vi "niDTS BT INSTR TX UTIL Average Type.vi"(7 "Type In":enum16{"RMS", "LOG", "SCALAR", "MAX", "MIN"}(ring)) -> (8 "Type Out":enum16{"RMS", "LOG", "SCALar", "MAX", "MIN"}(ring))   [LabVIEW 2015, in "niDTS BT.lvlib" / "niDTS BT INSTR TX.lvclass"]
uses:
  niDTS BT INSTR TX.lvclass
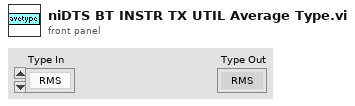
[diagram p1: front panel]
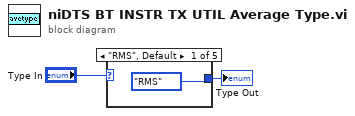
[diagram p0: block diagram]
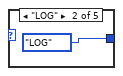
[diagram p2: hidden frame]
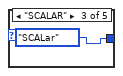
[diagram p3: hidden frame]
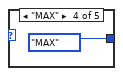
[diagram p4: hidden frame]
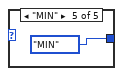
[diagram p5: hidden frame]
diagram:
  n1 = case shown="\"RMS\", Default" "Type In" {
    tunnel: [enum16{"RMS", "LOG", "SCALar", "MAX", "MIN"}."RMS" ("CONFigure:RFSA:BLUetooth:MEASurement:TXPower:AVERage:TxpAverageType") enum16{"RMS", "LOG", "SCALar", "MAX", "MIN"}."LOG" ("CONFigure:RFSA:BLUetooth:MEASurement:TXPower:AVERage:TxpAverageType") enum16{"RMS", "LOG", "SCALar", "MAX", "MIN"}."SCALar" ("CONFigure:RFSA:BLUetooth:MEASurement:TXPower:AVERage:TxpAverageType") enum16{"RMS", "LOG", "SCALar", "MAX", "MIN"}."MAX" ("CONFigure:RFSA:BLUetooth:MEASurement:TXPower:AVERage:TxpAverageType") enum16{"RMS", "LOG", "SCALar", "MAX", "MIN"}."MIN" ("CONFigure:RFSA:BLUetooth:MEASurement:TXPower:AVERage:TxpAverageType")] -> w1
    frame "RMS", Default {
    }
    frame "LOG" {
    }
    frame "SCALAR" {
    }
    frame "MAX" {
    }
    frame "MIN" {
    }
  }
  "Type Out" <- w1
